vi "Find FTDI Device.vi"(8 "error in (no error)":errorcluster, 11 "FTDI Serial Number":string) -> (0 "error out":errorcluster, 3 "VISA resource name":refnum<visa-resource-name>)   [LabVIEW 2020, in "FTDI Finder.lvlib"]
doc: "This VI will find the com port for the FTDI specified.\n\nCopyright 2021 JME Test Solutionc LLC\n\nwww.jmetestsolutions.com"
uses:
  FTDI Finder.lvlib
  <vilib>/registry/registry.llb/Registry SAM.ctl
  <vilib>/Instr/_visa.llb/VISA Find Search Mode.ctl
  <vilib>/regexp/Match Regular Expression.xnode
  <vilib>/registry/registry.llb/Read Registry Value Simple STR.vi
panel:
  out "Serial Numbers":string[](array[string])
  out "COM Ports":string[](array[string])
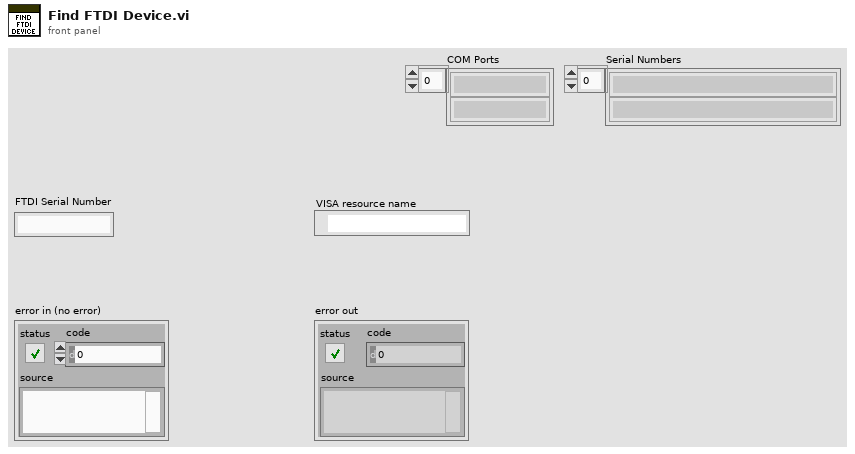
[diagram p1: front panel]
types:
  T1 = typedef "Registry SAM.ctl" = enum32{"KEY_QUERY_VALUE", "KEY_SET_VALUE", "KEY_CREATE_SUB_KEY", "KEY_ENUMERATE_SUB_KEYS", "KEY_NOTIFY", "KEY_CREATE_LINK", "KEY_READ", "KEY_WRITE", "KEY_ALL_ACCESS", "KEY_READ | KEY_WRITE"}
  T2 = typedef "Registry refnum.ctl" = refnum<k1>
  T3 = cluster{"numSubKeys":i32, "maxSubKeyLen":i32, "maxSubKeyClassLen":i32}
  T4 = typedef "VISA Find Search Mode.ctl" = u32
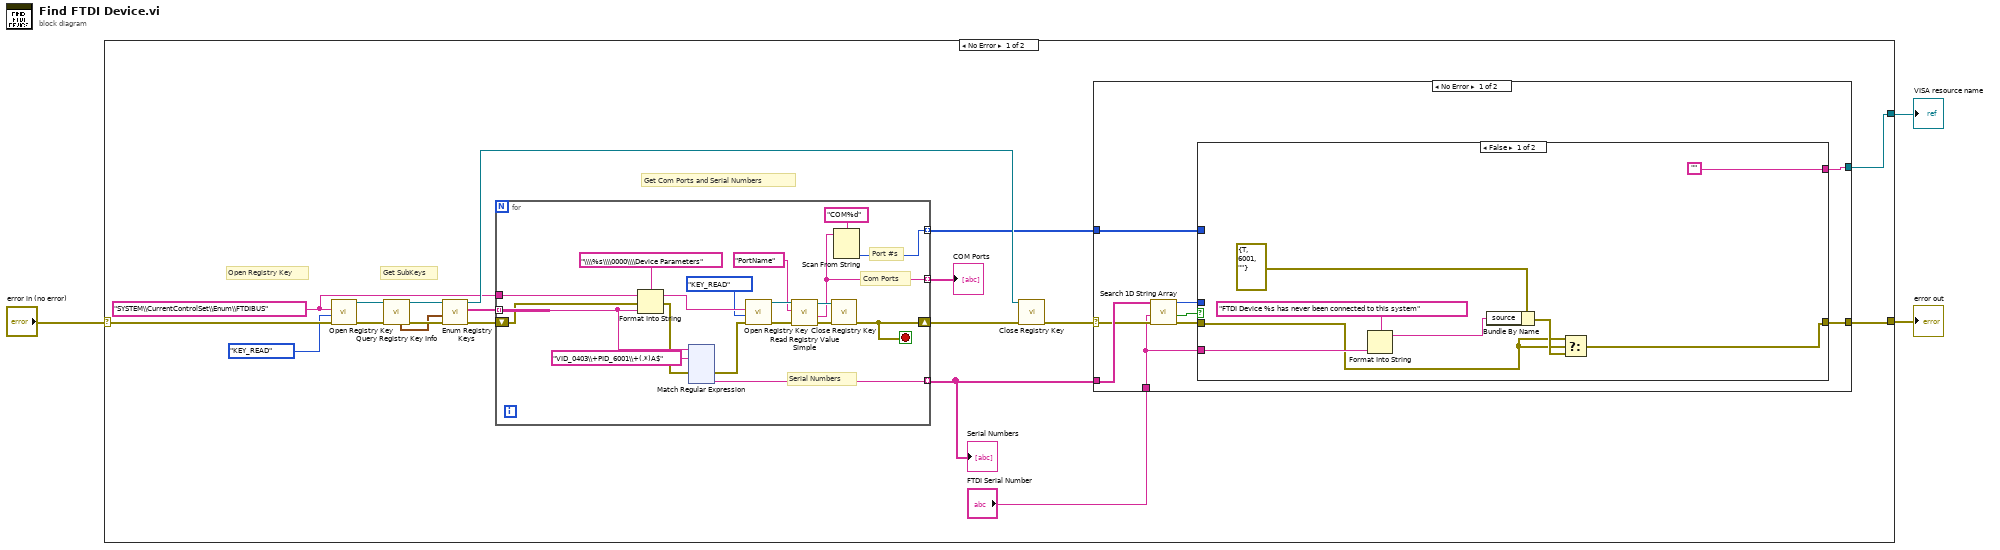
[diagram p0: block diagram]
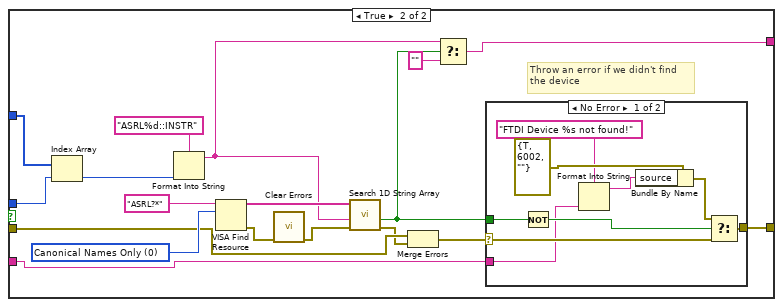
[diagram p2: hidden frame]
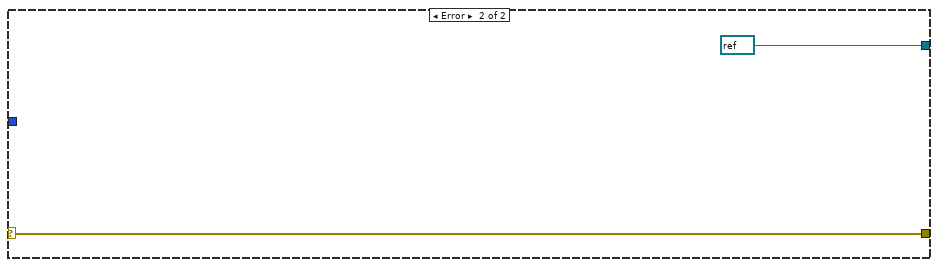
[diagram p4: hidden frame]
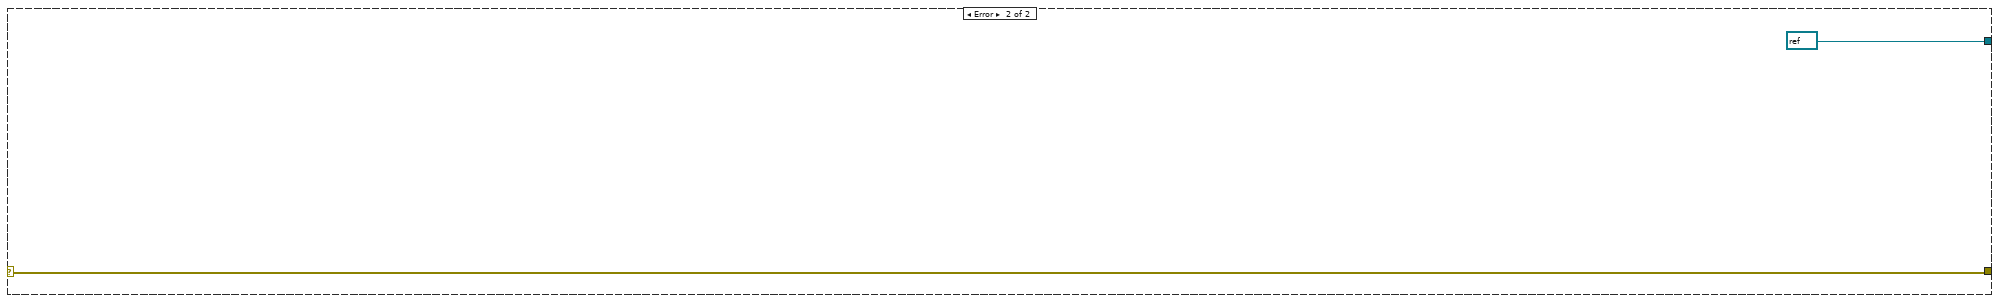
[diagram p5: hidden frame]
diagram:
  n1 = case shown="No Error" "error in (no error)" {
    selector: "error in (no error)" -> [w22 w206]
    tunnel: [w9 w206] -> w2
    tunnel: [w4 refnum<visa-resource-name> refnum ("VISA resource name")] -> w1
    frame No Error {
      w11 = "SYSTEM\\CurrentControlSet\\Enum\\FTDIBUS" ("subkey")
      # "Get Com Ports and Serial Numbers"
      # "Get SubKeys"
      # "Open Registry Key"
      n2 = call <vilib>:"Open Registry Key.vi"("error in (no error)"=w22, "security access mask (KEY_READ | KEY_WRITE)"=Registry_SAM."KEY_READ", "subkey"=w11) -> ("error out"=w19:errorcluster, "refnum out"=w20:T2)  [unwired: 7 in]
      n3 = call <vilib>:"Query Registry Key Info.vi"("error in (no error)"=w19, "refnum"=w20) -> ("error out"=w17:errorcluster, "refnum out"=w18:T2, "subkey info"=w16:T3)  [unwired: 5 in, 2 out]
      n4 = call <vilib>:"Enum Registry Keys.vi"("error in (no error)"=w17, "subkey info"=w16, "refnum"=w18) -> ("error out"=w15:errorcluster, "subkeys"=w12:string[], "refnum out"=w13:T2)  [unwired: 6 in]
      n5 = for {
        shift-right: [w81] -> w14
        shift-left: w15 -> [w79]
        tunnel: w12 -> [w80] mode=indexing
        tunnel: w11 -> [w88]
        tunnel: [w72] -> w10 mode=indexing
        tunnel: [w75] -> w6 mode=indexing
        tunnel: [w70] -> w5 mode=indexing
        stop <- w81 stop-if-true
        # "Port #s"
        # "Serial Numbers"
        # "Com Ports"
        n6 = Format Into String(format string="\\\\%s\\\\0000\\\\Device Parameters", initial string=w88, error in=w79, w80) -> (resulting string=w86:string, error out=w78:errorcluster)
        n7 = xnode "Match Regular Expression"("input string"=w80, "regular expression"="VID_0403\\+PID_6001\\+(.*)A$", "error in"=w78) -> ("error out"=w77:errorcluster, "submatch 1"=w75:string)  [unwired: 3 in, 4 out]
        n8 = call <vilib>:"Open Registry Key.vi"("error in (no error)"=w77, "security access mask (KEY_READ | KEY_WRITE)"=Registry_SAM."KEY_READ", "subkey"=w86) -> ("error out"=w85:errorcluster, "refnum out"=w84:T2)  [unwired: 7 in]
        n9 = call-poly <vilib>:"Read Registry Value Simple.vi"("error in (no error)"=w85, "value"="PortName", "refnum"=w84) -> ("error out"=w82:errorcluster, "String/Binary data"=w72:string, "refnum out"=w83:T2)  [unwired: 3 in, 1 out]
        n10 = call <vilib>:"Close Registry Key.vi"("error in (no error)"=w82, "refnum"=w83) -> ("error out"=w81:errorcluster)  [unwired: 5 in]
        n11 = Scan From String(format string="COM%d", input string=w72) -> (output 1=w70:i32)  [unwired: 3 in, 3 out]
      }
      "COM Ports" <- w10
      "Serial Numbers" <- w6
      n12 = call <vilib>:"Close Registry Key.vi"("error in (no error)"=w14, "refnum"=w13) -> ("error out"=w8:errorcluster)  [unwired: 5 in]
      n13 = case shown="No Error" w8 {
        selector: w8 -> [w29 w69]
        tunnel: [w31 w69] -> w9
        tunnel: "FTDI Serial Number" -> [w24 _]
        tunnel: w6 -> [w30 _]
        tunnel: w5 -> [w25 _]
        tunnel: [w23 refnum<visa-resource-name> refnum ("VISA resource name")] -> w4
        frame No Error {
          n14 = call "Search 1D String Array.vi"("error in (no error)"=w29, "Search String"=w24, "1D String Array"=w30) -> ("error out"=w27:errorcluster, "Found?"=w28:bool, "Index"=w26:i32)  [unwired: 6 in]
          n15 = case shown="False" w28 {
            tunnel: [w34 w45] -> w31
            tunnel: w27 -> [w33 w48]
            tunnel: w26 -> [_ w55]
            tunnel: w25 -> [_ w56]
            tunnel: w24 -> [w39 w44]
            tunnel: ["" w41] -> w23
            frame False {
              n16 = Format Into String(format string="FTDI Device %s has never been connected to this system", w39) -> (resulting string=w36:string)  [unwired: 2 in, 1 out]
              n17 = Bundle By Name(cluster=errorcluster {"status"=TRUE, "code"=6001, "source"=""} ("error out"), "source"=w36) -> (w35:errorcluster)
              n18 = Select(t=w33, s=w33, f=w35) -> (s? t:f=w34:errorcluster)
            }
            frame True {
              w57 = T4 0 items=["Canonical Names Only"=0, "Aliases Only"=2, "Include Matching Aliases"=3, "Include All Aliases"=4] ("Search Mode")
              # "Throw an error if we didn't find\nthe device"
              n19 = Index Array(array=w56, index=w55) -> (element=w54:i32)
              n20 = Format Into String(format string="ASRL%d::INSTR", w54) -> (resulting string=w42:string)  [unwired: 2 in, 1 out]
              n21 = VISA Find Resource(10:w57, 11:"ASRL?*" ("expression (\"?*\")")) -> (0:w50:errorcluster, 3:w51:string[])  [unwired: 1 in, 1 out]
              n22 = call <vilib>:"Clear Errors.vi"("error in (no error)"=w50) -> ("error out"=w49:errorcluster)  [unwired: 5 in, 1 out]
              n23 = call "Search 1D String Array.vi"("error in (no error)"=w49, "Search String"=w42, "1D String Array"=w51) -> ("error out"=w47:errorcluster, "Found?"=w43:bool)  [unwired: 6 in, 1 out]
              n24 = Merge Errors(w48, w47) -> (w46:errorcluster)
              n25 = Select(t=w42, s=w43, f="") -> (s? t:f=w41:string)
              n26 = case shown="No Error" w46 {
                selector: w46 -> [w64 w67]
                tunnel: [w63 w67] -> w45
                tunnel: w43 -> [w66 _]
                tunnel: w44 -> [w59 _]
                frame No Error {
                  n27 = Not(x=w66) -> (.not. x?=w65:bool)
                  n28 = Format Into String(format string="FTDI Device %s not found!", w59) -> (resulting string=w60:string)  [unwired: 2 in, 1 out]
                  n29 = Bundle By Name(cluster=errorcluster {"status"=TRUE, "code"=6002, "source"=""} ("error out"), "source"=w60) -> (w61:errorcluster)
                  n30 = Select(t=w61, s=w65, f=w64) -> (s? t:f=w63:errorcluster)
                }
                frame Error {
                }
              }
            }
          }
        }
        frame Error {
        }
      }
    }
    frame Error {
    }
  }
  "error out" <- w2
  "VISA resource name" <- w1
